vi "Sig0.vi"(3 "x":u64) -> (1 "Sig0":u64)   [LabVIEW 2020, in "NI_SHA-512.lvclass"]
doc: "Computes the SHA-2 \\Sigma_0(x) function."
uses:
  <vilib>/security/Message Digest/SHA-2/SHA-512/NI_SHA-512.lvclass
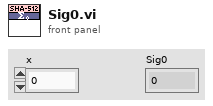
[diagram p1: front panel]
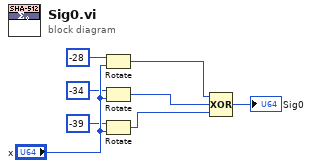
[diagram p0: block diagram]
diagram:
  n1 = Rotate(1:"x", 2:i16 -28 ("y")) -> (0:w1:u64)
  n2 = Rotate(1:"x", 2:i16 -34 ("y")) -> (0:w2:u64)
  n3 = Rotate(1:"x", 2:i16 -39 ("y")) -> (0:w3:u64)
  n4 = Compound Arithmetic op=XOR(w1, w2, w3) -> (→"Sig0":u64)
